vi "TestColores.vi"() -> ()   [LabVIEW 2017]
panel:
  in  "Numeric Control":dbl
  in  "Numeric":dbl
  in  "Color Box 2":u32(colorbox)
  in  "Color Box":u32(colorbox)
  in  "stop":bool
  out "Numeric Text.Text Colors:Text Color":u32 format="%x"
  in  "Target X(T)":dbl min=-0.5 max=0.5 step=0.001 format="%.2f"
  in  "Numeric 2":dbl
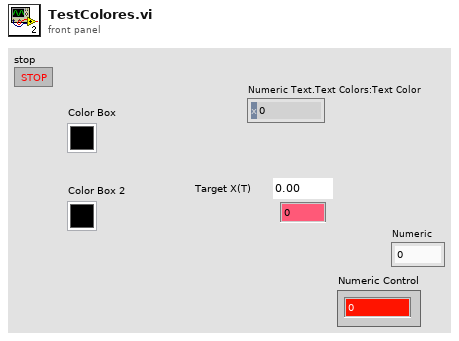
[diagram p1: front panel]
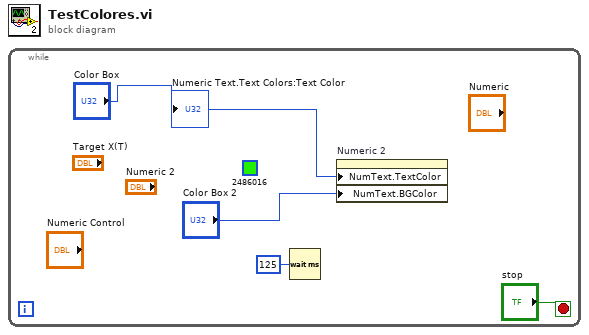
[diagram p0: block diagram]
diagram:
  n1 = while {
    stop <- "stop" stop-if-true
    (unwired) u32 2486016 ("Color Box 2")
    n2 = Wait (ms)(milliseconds to wait=u32 125) -> ()  [unwired: 1 out]
    n3 = property on="Numeric 2" class="DigNum (strict)"("NumText.TextColor"="Color Box", "NumText.BGColor"="Color Box 2") -> ()  [unwired: 2 in, 2 out]
    "Numeric Text.Text Colors:Text Color" <- "Color Box"
  }
